vi "4.循环计时器.vi"() -> ()   [LabVIEW 2019]
uses:
  <vilib>/rvi/Emulation/niFpgaGetClockAttributes.vi
  <vilib>/rvi/Emulation/niFpgaSctlEmulationGetInTimedLoop.vi
  <vilib>/rvi/Emulation/niFpgaEmulationReportErrorSimple.vi
  <vilib>/rvi/eio/common/nirviEmuTemplateMethod_errors.vi
  <vilib>/rvi/Emulation/niFpgaCriticalErrorInLSC.vi
  <vilib>/eio/EIONode/EIONode.xnode
panel:
  in  "阈值":fxp<+/-,24,5>=3.0
  out "ConnectorA/AI0":fxp<+/-,24,5>
  in  "Count(uSec) 2":u16=200 caption="计数器(uSec)"
  in  "ConnectorA/AO0":i16(slide) scale=1.0..5.0
  in  "Count(uSec)":u16=100 caption="计数器(uSec)"
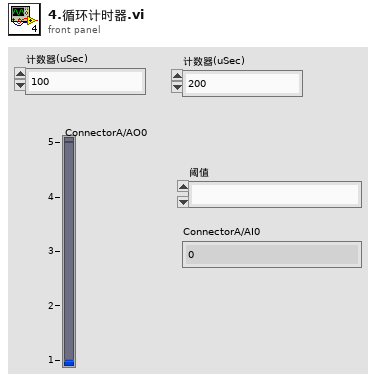
[diagram p1: front panel]
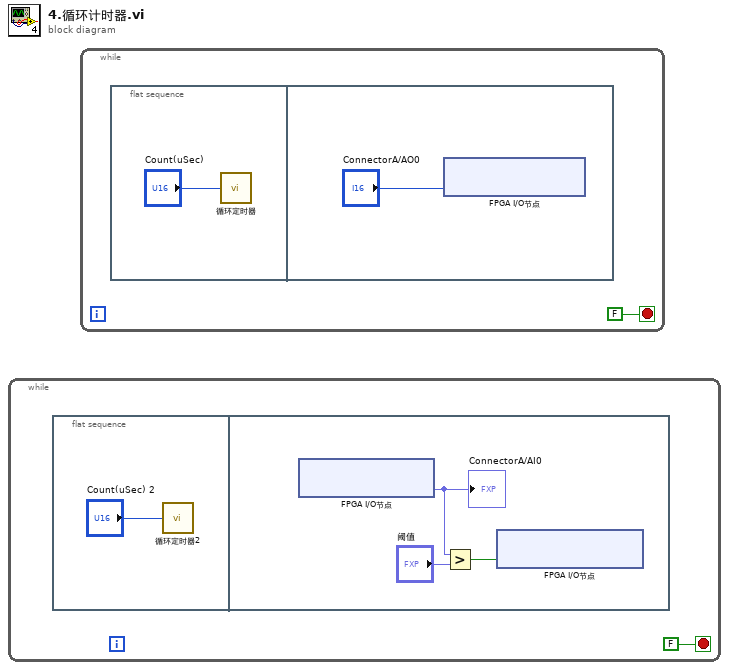
[diagram p0: block diagram]
diagram:
  n1 = while {
    stop <- FALSE stop-if-true
    n2 = flat-sequence {
      frame #0 {
        n3 = call "循环定时器2"("Count(uSec)"="Count(uSec) 2") -> ()  [unwired: 1 out]
      }
      frame #1 {
        n4 = xnode "FPGA I/O节点"() -> ("ConnectorA/AI0"=w5:fxp<+/-,24,5>)  [unwired: 1 in, 1 out]
        "ConnectorA/AI0" <- w5
        n5 = Greater?(x=w5, y="阈值") -> (0:w3:bool)
        n6 = xnode "FPGA I/O节点"("ConnectorA/DIO0"=w3) -> ()  [unwired: 1 in, 1 out]
      }
    }
  }
  n7 = while {
    stop <- FALSE stop-if-true
    n8 = flat-sequence {
      frame #0 {
        n9 = call "循环定时器"("Count(uSec)"="Count(uSec)") -> ()  [unwired: 1 out]
      }
      frame #1 {
        n10 = xnode "FPGA I/O节点"("ConnectorA/AO0"="ConnectorA/AO0") -> ()  [unwired: 1 in, 1 out]
      }
    }
  }
